vi "SimpleGetPeaksExample.vi"() -> ()   [LabVIEW 2016]
doc: "This example VI demonstrates the use of the #GetPeaks command to retrieve peaks data from Hyperion instruments."
uses:
  h.Library/ACQ/CTL/h.ACQ.PeaksData.ctl
  h.Library/ACQ/CTL/h.ACQ.PeaksWvl.ctl
  h.Library.lvlib
panel:
  out "Peaks Data":T1 {"Peaks Wvls, nm"."Peak Wvls, nm" format="%#_8g"}
  in  "Address":string="10.0.0.55"
  # "Hyperion Simple #GetPeaks Example"
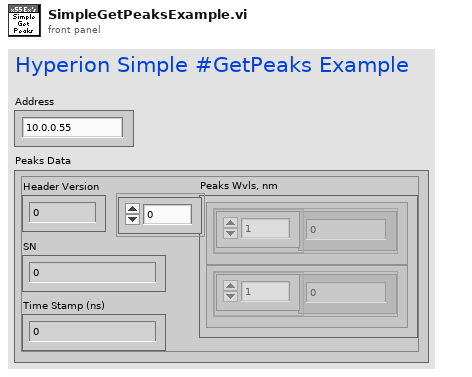
[diagram p1: front panel]
types:
  T1 = typedef "h.Library.lvlib/h.ACQ.PeaksData.ctl" = cluster{"SN":u64, "Time Stamp (ns)":u64, "Header Version":u16, "Peaks Wvls, nm":T2[]}
  T2 = typedef "h.Library.lvlib/h.ACQ.PeaksWvl.ctl" = cluster{"Peak Wvls, nm":dbl[]}
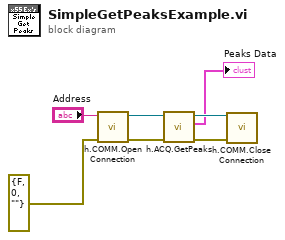
[diagram p0: block diagram]
diagram:
  n1 = call "h.COMM.Open Connection.vi"("error in"=errorcluster {"status"=FALSE, "code"=0, "source"=""}, "Address"="Address") -> ("error out"=w3:errorcluster, "Connection ID"=w5:refnum<k5>)  [unwired: 8 in]
  n2 = call "h.ACQ.GetPeaks.vi"("error in"=w3, "Connection ID In"=w5) -> ("error out"=w2:errorcluster, "Peaks Data"=→"Peaks Data":T1, "Connection ID Out"=w4:refnum<k5>)  [unwired: 7 in]
  n3 = call "h.COMM.Close Connection.vi"("error in"=w2, "Connection ID"=w4) -> ()  [unwired: 9 in, 1 out]
